vi "CRYSort Calibration 2D.vi"(11 "Calibration In":T1 {"Calibration 2D"."Sens Curve"."Z data" items=["dB", "Lin"]; "Calibration 2D"."Sens Curve"."X data" items=["dB", "Lin"]; "Calibration 2D"."Sens Curve"."Y data" items=["dB", "Lin"]; "Calibration 2D"."Sens Curve"."Z dB ref" format="%.1f"; "Calibration 2D"."Sens Curve"."Z axis" items=["Log", "Lin"]; "Calibration 2D"."Sens Curve"."X dB ref" format="%.1f"; "Calibration 2D"."Sens Curve"."X axis" items=["Log", "Lin"]; "Calibration 2D"."Sens Curve"."Y axis" items=["Log", "Lin"]; "Calibration 2D"."Sens Curve"."Y dB ref" format="%.1f"; "Calibration 2D"."Sens Curve"."Curve"."z" format="%.2f"; "Calibration 2D"."Sens Curve"."Curve"."y" format="%.2f"; "Calibration 2D"."Sens Curve"."Curve"."x" format="%.2f"; "Calibration 2D"."EQ Curve"."Z data" items=["dB", "Lin"]; "Calibration 2D"."EQ Curve"."X data" items=["dB", "Lin"]; "Calibration 2D"."EQ Curve"."Y data" items=["dB", "Lin"]; "Calibration 2D"."EQ Curve"."Z dB ref" format="%.1f"; "Calibration 2D"."EQ Curve"."Z axis" items=["Log", "Lin"]; "Calibration 2D"."EQ Curve"."X dB ref" format="%.1f"; "Calibration 2D"."EQ Curve"."X axis" items=["Log", "Lin"]; "Calibration 2D"."EQ Curve"."Y axis" items=["Log", "Lin"]; "Calibration 2D"."EQ Curve"."Y dB ref" format="%.1f"; "Calibration 2D"."EQ Curve"."Curve"."z" format="%.2f"; "Calibration 2D"."EQ Curve"."Curve"."y" format="%.2f"; "Calibration 2D"."EQ Curve"."Curve"."x" format="%.2f"; "Calibration 2D"."Corr Curve"."Z data" items=["dB", "Lin"]; "Calibration 2D"."Corr Curve"."X data" items=["dB", "Lin"]; "Calibration 2D"."Corr Curve"."Y data" items=["dB", "Lin"]; "Calibration 2D"."Corr Curve"."Z dB ref" format="%.1f"; "Calibration 2D"."Corr Curve"."Z axis" items=["Log", "Lin"]; "Calibration 2D"."Corr Curve"."X dB ref" format="%.1f"; "Calibration 2D"."Corr Curve"."X axis" items=["Log", "Lin"]; "Calibration 2D"."Corr Curve"."Y axis" items=["Log", "Lin"]; "Calibration 2D"."Corr Curve"."Y dB ref" format="%.1f"; "Calibration 2D"."Corr Curve"."Curve"."z" format="%.2f"; "Calibration 2D"."Corr Curve"."Curve"."y" format="%.2f"; "Calibration 2D"."Corr Curve"."Curve"."x" format="%.2f"; "Calibration 2D"."Calibration"."EQ Step size" items=["R10", "R20", "R40", "R80", "User"]; "Calibration 2D"."Calibration"."Corr Step size" items=["R10", "R20", "R40", "R80", "User"]}) -> (3 "Calibration Out":T1 {"Calibration 2D"."Sens Curve"."Z data" items=["dB", "Lin"]; "Calibration 2D"."Sens Curve"."X data" items=["dB", "Lin"]; "Calibration 2D"."Sens Curve"."Y data" items=["dB", "Lin"]; "Calibration 2D"."Sens Curve"."Z dB ref" format="%.1f"; "Calibration 2D"."Sens Curve"."Z axis" items=["Log", "Lin"]; "Calibration 2D"."Sens Curve"."X dB ref" format="%.1f"; "Calibration 2D"."Sens Curve"."X axis" items=["Log", "Lin"]; "Calibration 2D"."Sens Curve"."Y axis" items=["Log", "Lin"]; "Calibration 2D"."Sens Curve"."Y dB ref" format="%.1f"; "Calibration 2D"."Sens Curve"."Curve"."z" format="%.2f"; "Calibration 2D"."Sens Curve"."Curve"."y" format="%.2f"; "Calibration 2D"."Sens Curve"."Curve"."x" format="%.2f"; "Calibration 2D"."EQ Curve"."Z data" items=["dB", "Lin"]; "Calibration 2D"."EQ Curve"."X data" items=["dB", "Lin"]; "Calibration 2D"."EQ Curve"."Y data" items=["dB", "Lin"]; "Calibration 2D"."EQ Curve"."Z dB ref" format="%.1f"; "Calibration 2D"."EQ Curve"."Z axis" items=["Log", "Lin"]; "Calibration 2D"."EQ Curve"."X dB ref" format="%.1f"; "Calibration 2D"."EQ Curve"."X axis" items=["Log", "Lin"]; "Calibration 2D"."EQ Curve"."Y axis" items=["Log", "Lin"]; "Calibration 2D"."EQ Curve"."Y dB ref" format="%.1f"; "Calibration 2D"."EQ Curve"."Curve"."z" format="%.2f"; "Calibration 2D"."EQ Curve"."Curve"."y" format="%.2f"; "Calibration 2D"."EQ Curve"."Curve"."x" format="%.2f"; "Calibration 2D"."Corr Curve"."Z data" items=["dB", "Lin"]; "Calibration 2D"."Corr Curve"."X data" items=["dB", "Lin"]; "Calibration 2D"."Corr Curve"."Y data" items=["dB", "Lin"]; "Calibration 2D"."Corr Curve"."Z dB ref" format="%.1f"; "Calibration 2D"."Corr Curve"."Z axis" items=["Log", "Lin"]; "Calibration 2D"."Corr Curve"."X dB ref" format="%.1f"; "Calibration 2D"."Corr Curve"."X axis" items=["Log", "Lin"]; "Calibration 2D"."Corr Curve"."Y axis" items=["Log", "Lin"]; "Calibration 2D"."Corr Curve"."Y dB ref" format="%.1f"; "Calibration 2D"."Corr Curve"."Curve"."z" format="%.2f"; "Calibration 2D"."Corr Curve"."Curve"."y" format="%.2f"; "Calibration 2D"."Corr Curve"."Curve"."x" format="%.2f"; "Calibration 2D"."Calibration"."EQ Step size" items=["R10", "R20", "R40", "R80", "User"]; "Calibration 2D"."Calibration"."Corr Step size" items=["R10", "R20", "R40", "R80", "User"]})   [LabVIEW 2013]
uses:
  Typedef Control/CRYCalibration All Cluster.ctl
  Typedef Control/CRYCalibration 2DCluster.ctl
  Typedef Control/CRYCalibration Cluster.ctl
  Typedef Control/CRYData Cluster.ctl
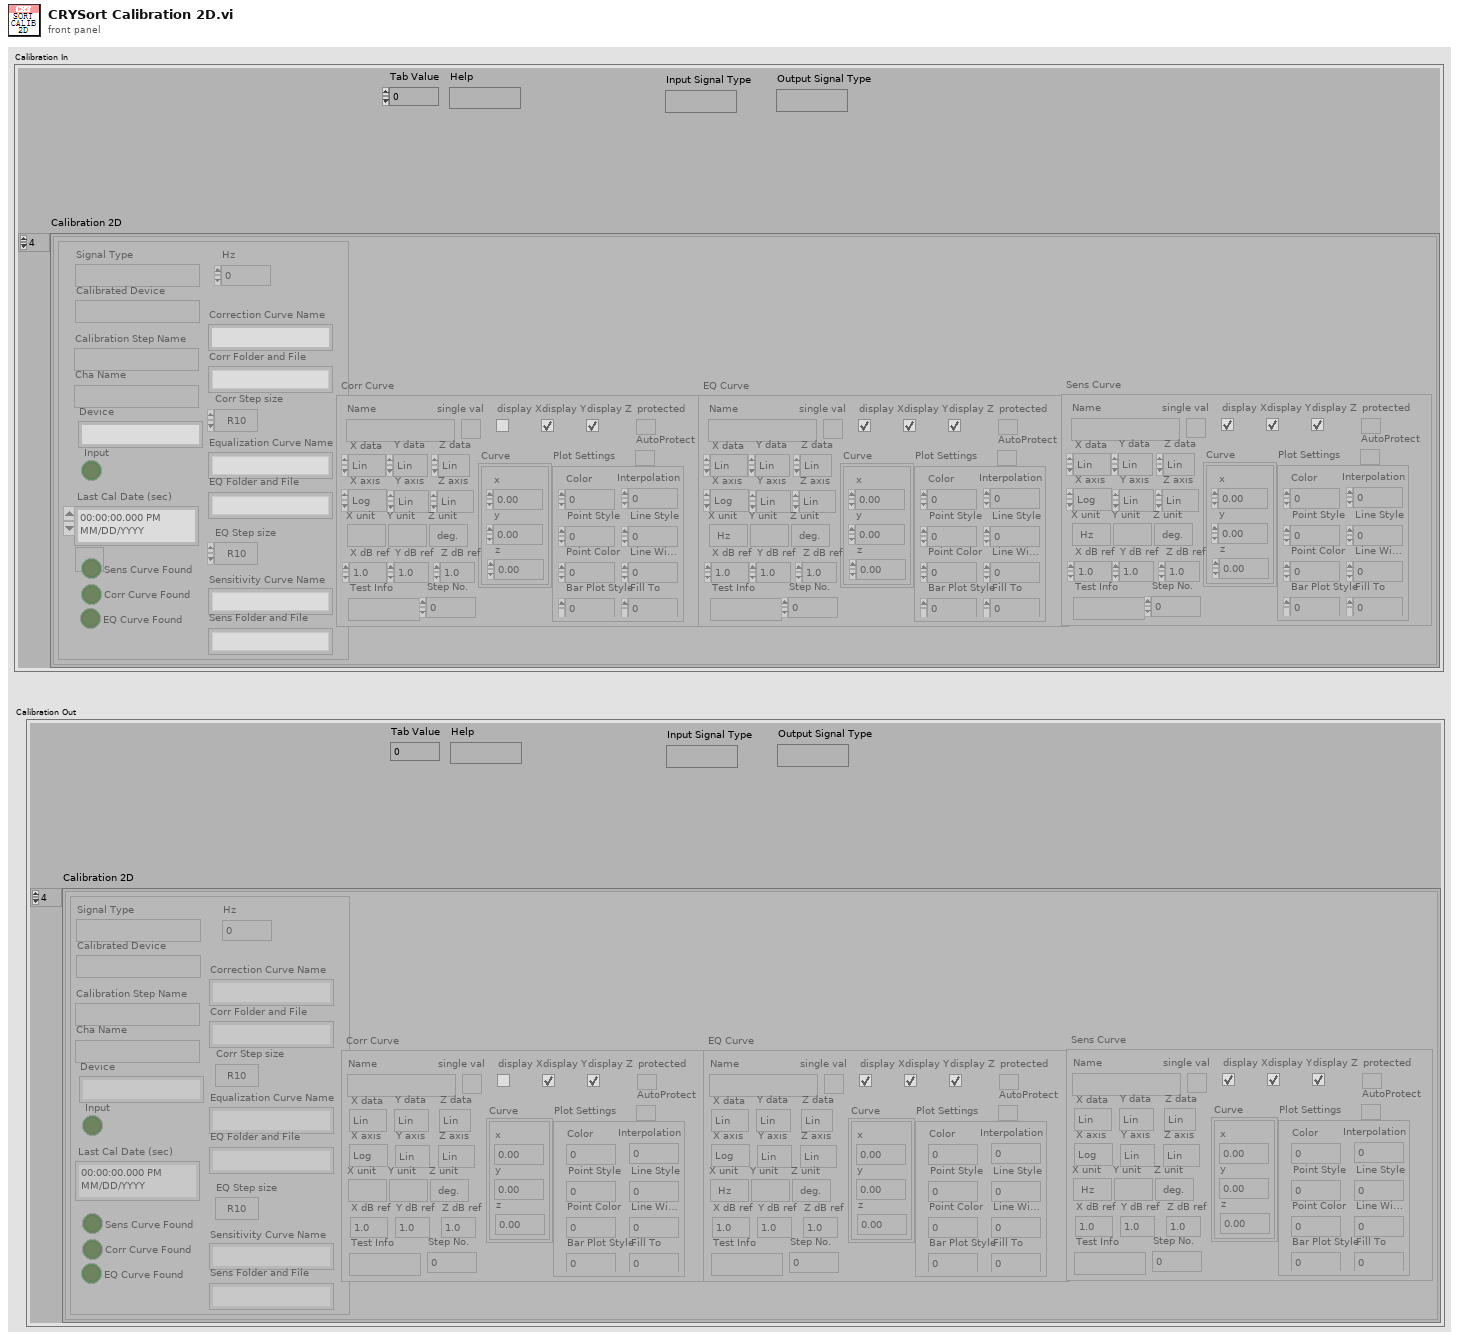
[diagram p1: front panel]
types:
  T1 = typedef "CRYCalibration All Cluster.ctl" = cluster{"Calibration 2D":T2[], "Help":string, "Tab Value":i32, "Input Signal Type":string, "Output Signal Type":string}
  T2 = typedef "CRYCalibration 2DCluster.ctl" = cluster{"Calibration":T3, "Corr Curve":T4, "EQ Curve":T4, "Sens Curve":T4}
  T3 = typedef "CRYCalibration Cluster.ctl" = cluster{"Calibration Step Name":string, "Device":string, "Correction Curve Name":string, "Equalization Curve Name":string, "Sensitivity Curve Name":string, "Corr Folder and File":string, "EQ Folder and File":string, "Sens Folder and File":string, "Corr Step size":u16, "EQ Step size":u16, "Input":bool, "Last Cal Date (sec)":timestamp, "Cha Name":string, "Corr Curve Found":bool, "EQ Curve Found":bool, "Sens Curve Found":bool, "Signal Type":string, "Calibrated Device":string, "Hz":u32}
  T4 = typedef "CRYData Cluster.ctl" = cluster{"Name":string, "Curve":cluster{"x":dbl, "y":dbl, "z":dbl}[], "X data":u16, "Y data":u16, "Z data":u16, "X axis":u16, "Y axis":u16, "Z axis":u16, "X unit":string, "Y unit":string, "Z unit":string, "X dB ref":dbl, "Y dB ref":dbl, "Z dB ref":dbl, "single val":bool, "protected":bool, "display X":bool, "display Y":bool, "display Z":bool, "Test Info":string, "Step No.":i32, "Plot Settings":cluster{"Color":u32, "Interpolation":u8, "Point Style":u8, "Line Style":u8, "Point Color":u32, "Line Width":u8, "Bar Plot Style":u8, "Fill To":i16}, "AutoProtect":bool}
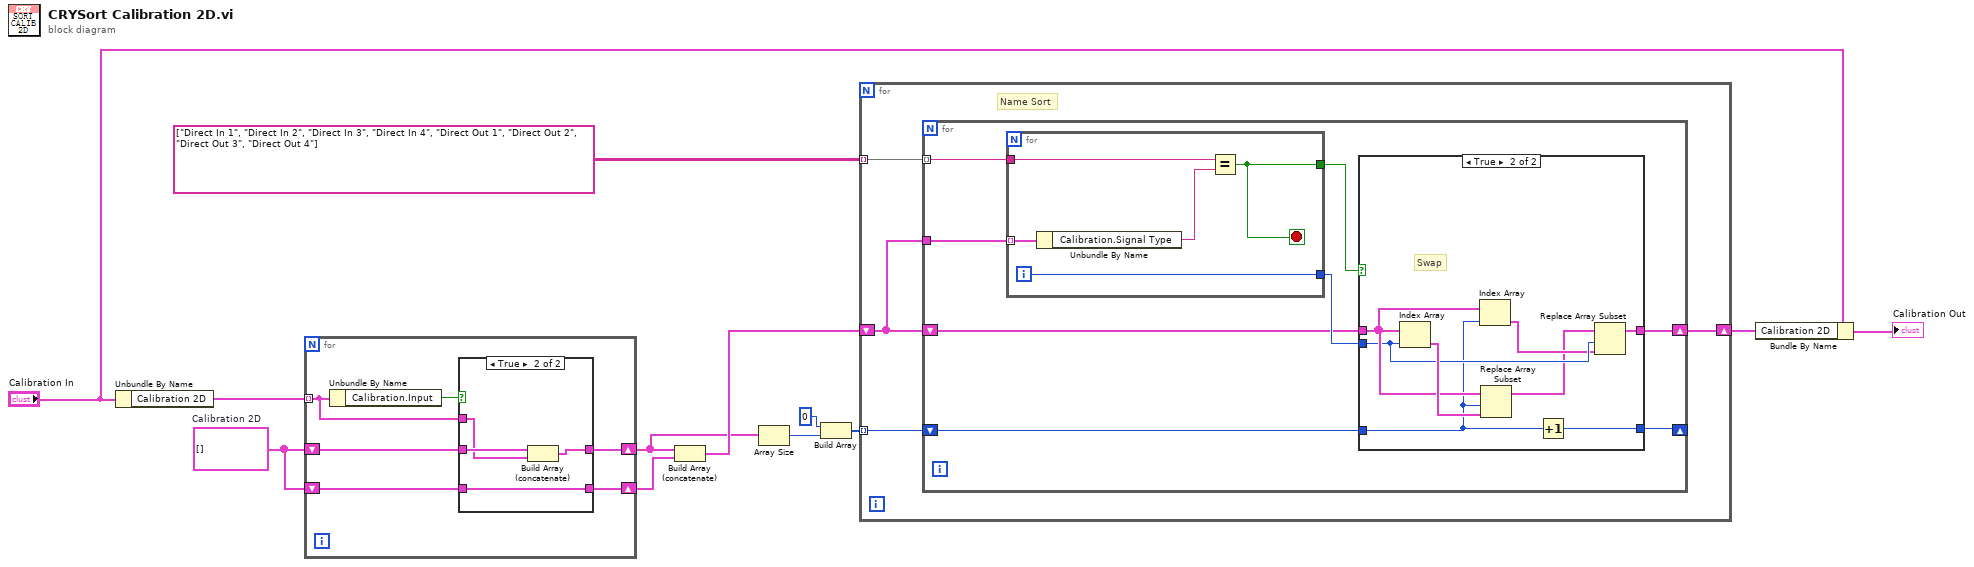
[diagram p0: block diagram]
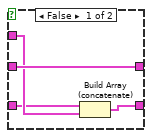
[diagram p2: hidden frame]
diagram:
  w7 = T2[] []  # Calibration 2D
  n1 = Unbundle By Name("Calibration In") -> ("Calibration 2D"=w8:T2[])
  n2 = for {
    tunnel: w8 -> [w14] mode=indexing
    shift-right: [w15] -> w2
    shift-left: w7 -> [w16]
    shift-right: [w13] -> w5
    shift-left: w7 -> [w17]
    n3 = Unbundle By Name(w14) -> ("Calibration.Input"=w18:bool)
    n4 = case shown="True" w18 {
      tunnel: w17 -> [w20 w23]
      tunnel: w16 -> [w22 w26]
      tunnel: [w22 w25] -> w15
      tunnel: w14 -> [w21 w24]
      tunnel: [w19 w23] -> w13
      frame False {
        n5 = Build Array (concatenate)(w20, w21) -> (w19:T2[])
      }
      frame True {
        n6 = Build Array (concatenate)(w26, w24) -> (w25:T2[])
      }
    }
  }
  n7 = Build Array (concatenate)(w2, w5) -> (w6:T2[])
  n8 = Array Size(array=w2) -> (size(s)=w4:i32)
  n9 = Build Array(0 ("element"), w4) -> (w1:i32[])
  n10 = for {
    tunnel: string[][] [["Direct In 1", "Direct In 2", "Direct In 3", "Direct In 4"], ["Direct Out 1", "Direct Out 2", "Direct Out 3", "Direct Out 4"]] -> [w29] mode=indexing
    shift-right: [w30] -> w12
    shift-left: w6 -> [w28]
    tunnel: w1 -> [w27] mode=indexing
    # "Name Sort"
    n11 = for {
      tunnel: w28 -> [w38]
      tunnel: w29 -> [w37] mode=indexing
      shift-right: [w33] -> w30
      shift-left: w28 -> [w34]
      shift-right: [w31] -> _
      shift-left: w27 -> [w32]
      n12 = for {
        tunnel: w38 -> [w53] mode=indexing
        tunnel: w37 -> [w52]
        tunnel: [w50] -> w36
        tunnel: [w49] -> w35
        i -> [w49]
        stop <- w50 stop-if-true
        n13 = Unbundle By Name(w53) -> ("Calibration.Signal Type"=w51:string)
        n14 = Equal?(x=w52, y=w51) -> (x = y?=w50:bool)
      }
      n15 = case shown="True" w36 {
        tunnel: w35 -> [_ w46]
        tunnel: w34 -> [w40 w47]
        tunnel: [w40 w43] -> w33
        tunnel: w32 -> [w39 w42]
        tunnel: [w39 w41] -> w31
        frame False {
        }
        frame True {
          # "Swap"
          n16 = Index Array(array=w47, index=w46) -> (element=w48:T2)
          n17 = Index Array(array=w47, index=w42) -> (element=w45:T2)
          n18 = Replace Array Subset(array=w47, new element=w48, index=w42) -> (w44:T2[])
          n19 = Increment(x=w42) -> (x+1=w41:i32)
          n20 = Replace Array Subset(array=w44, new element=w45, index=w46) -> (w43:T2[])
        }
      }
    }
  }
  n21 = Bundle By Name(cluster="Calibration In", "Calibration 2D"=w12) -> (→"Calibration Out":T1)
